vi "FlexDDS-NG_DCP_WriteCFR2_C.vi"(6 "FM gain (0..15)":u32 max=15 step=1, 8 "Digital ramp destination":enum32{"Frequency", "Phase", "Amplitude"}(ring), 9 "CFR2 bits":T1={"Enable ASF from STP (F)"=FALSE, "Digital ramp enable (F)"=FALSE, "Digital ramp no-dwell high (F)"=FALSE, "Digital ramp no-dwell low (F)"=FALSE, "Matched latency enable (T)"=TRUE, "Parallel data port enable (F)"=FALSE}, 10 "Channels":T2(ring)=enum."Both channels", 11 "initial instruction string":string) -> (3 "appended instruction string":string)   [LabVIEW 2016]
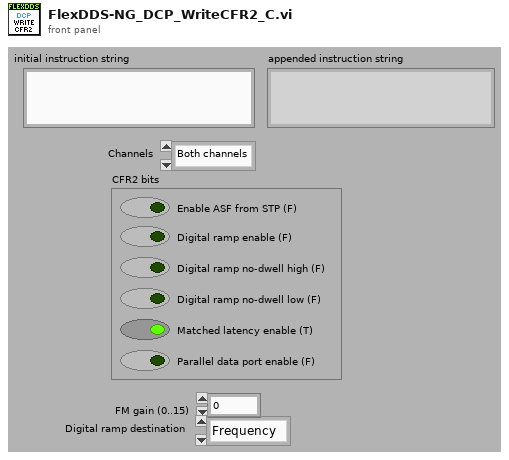
[diagram p1: front panel]
types:
  T1 = cluster{"Enable ASF from STP (F)":bool, "Digital ramp enable (F)":bool, "Digital ramp no-dwell high (F)":bool, "Digital ramp no-dwell low (F)":bool, "Matched latency enable (T)":bool, "Parallel data port enable (F)":bool}
  T2 = enum32{"Channel 0", "Channel 1", "Both channels"}
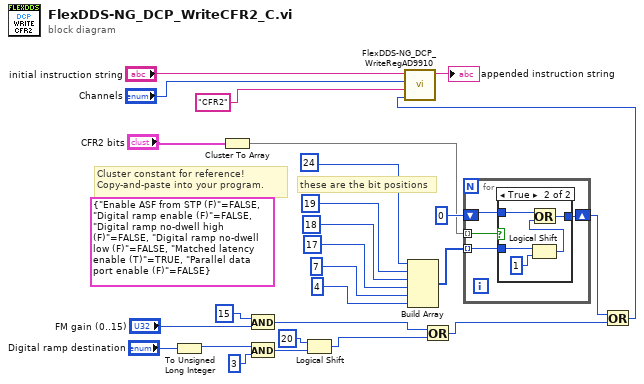
[diagram p0: block diagram]
diagram:
  (unwired) T1 {"Enable ASF from STP (F)"=FALSE, "Digital ramp enable (F)"=FALSE, "Digital ramp no-dwell high (F)"=FALSE, "Digital ramp no-dwell low (F)"=FALSE, "Matched latency enable (T)"=TRUE, "Parallel data port enable (F)"=FALSE} ("CFR2 bits")
  # "these are the bit positions"
  # "Cluster constant for reference!\nCopy-and-paste into your program."
  n1 = To Unsigned Long Integer(number="Digital ramp destination") -> (unsigned 32bit integer=w7:u32)
  n2 = Cluster To Array(cluster="CFR2 bits") -> (array=w13:bool[])
  n3 = And(x=u32 15, y="FM gain (0..15)") -> (x .and. y?=w3:u32)
  n4 = And(x=w7, y=u32 3) -> (x .and. y?=w5:u32)
  n5 = Logical Shift(y=i8 20, x=w5) -> (x << y=w2:u32)
  n6 = Build Array(24 ("single tone profile (0..7)"), 19 ("single tone profile (0..7)"), 18 ("single tone profile (0..7)"), 17 ("single tone profile (0..7)"), 7 ("single tone profile (0..7)"), 4 ("single tone profile (0..7)")) -> (w16:i32[])
  n7 = Or(x=w3, y=w2) -> (x .or. y?=w1:u32)
  n8 = for {
    tunnel: w13 -> [w27] mode=indexing
    tunnel: w16 -> [w30] mode=indexing
    shift-right: [w29] -> w12
    shift-left: u32 0 ("x") -> [w28]
    n9 = case shown="True" w27 {
      tunnel: w30 -> [_ w36]
      tunnel: [w31 w33] -> w29
      tunnel: w28 -> [w31 w32]
      frame False {
      }
      frame True {
        n10 = Logical Shift(y=w36, x=u32 1) -> (x << y=w34:u32)
        n11 = Or(x=w32, y=w34) -> (x .or. y?=w33:u32)
      }
    }
  }
  n12 = Or(x=w12, y=w1) -> (x .or. y?=w11:u32)
  n13 = call "FlexDDS-NG_DCP_WriteRegAD9910.vi"("register content"=w11, "AD9910 register name"="CFR2" ("format string"), "Channels"="Channels", "initial instruction string"="initial instruction string") -> ("appended instruction string"=→"appended instruction string":string)  [unwired: 7 in]
